vi "EFMC-7.vi"(0 "数组":u8[](array[numeric])) -> (1 "视速度增量":cluster{"X轴增量":i16, "Y轴增量":i16, "Z轴增量":i16}, 2 "姿态和速度增量有效性":T2, 3 "俯仰角速率":i16, 4 "滚转角速率":i16, 6 "角度增量":cluster{"X轴角增量":i16, "Y轴角增量":i16, "Z轴角增量":i16}, 8 "X轴过载":i16, 10 "偏航角速率":i16, 12 "Z轴过载":i16, 13 "角速率和过载有效性":T1, 14 "Y轴过载":i16)   [LabVIEW 2012]
uses:
  index-i16.vi
  XX-I16.vi
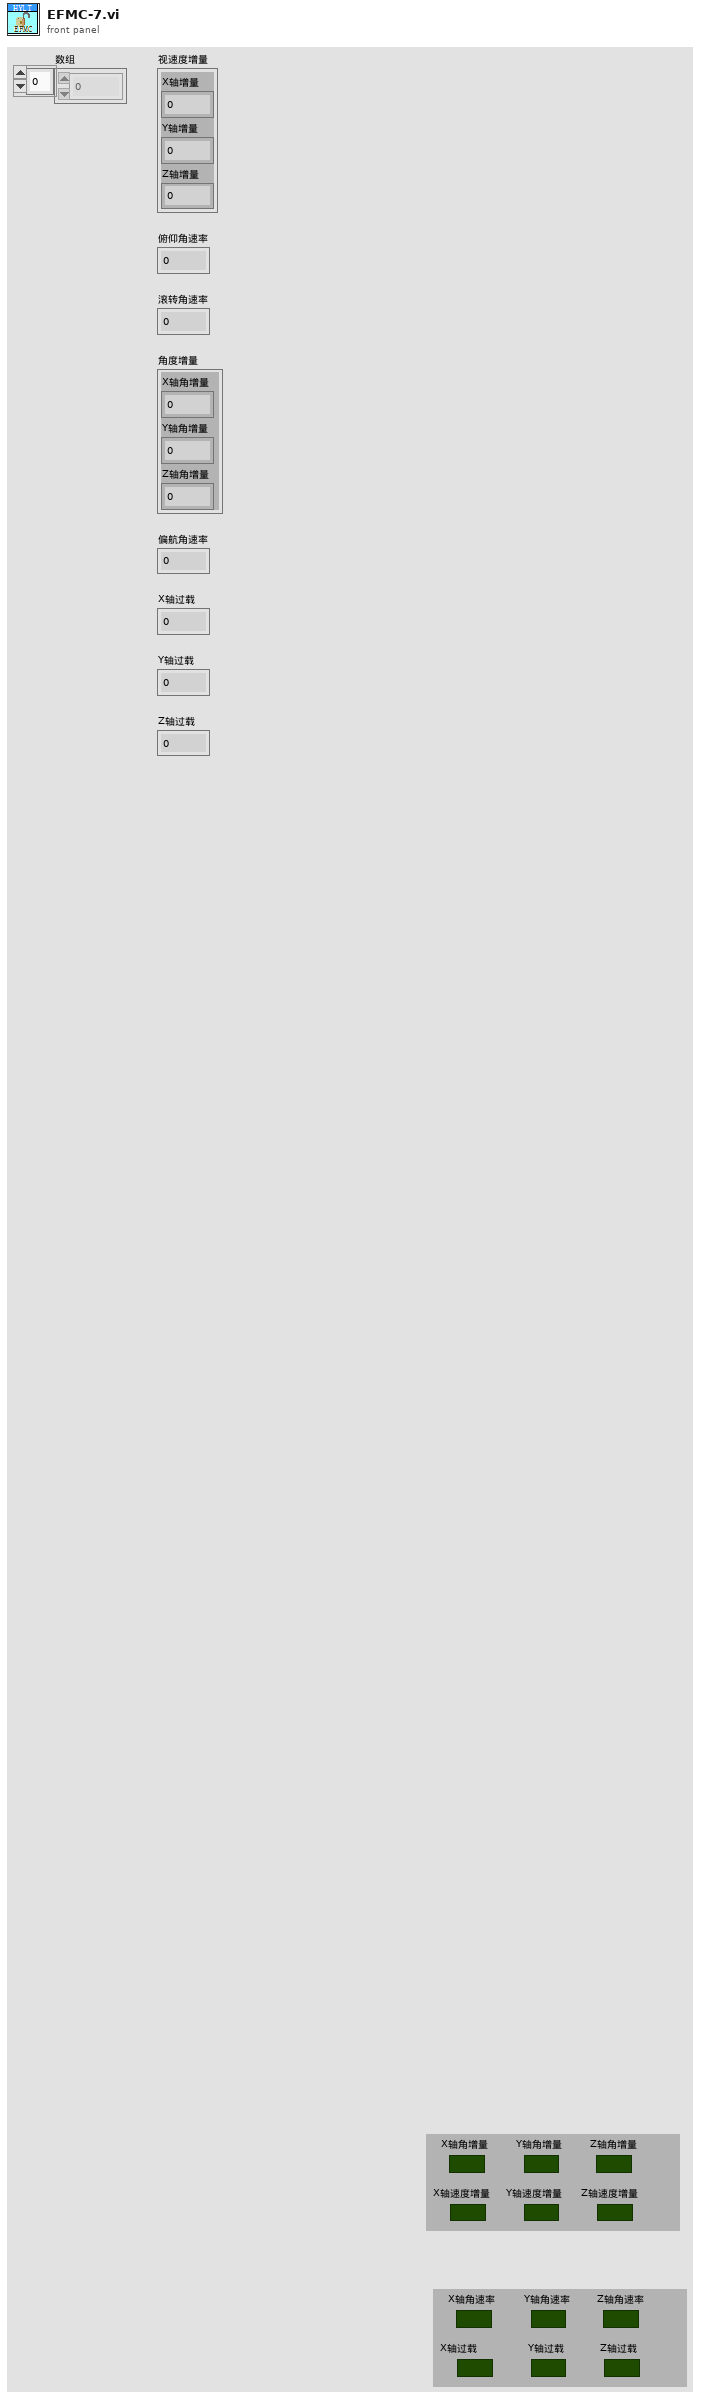
[diagram p1: front panel]
types:
  T1 = cluster{"X轴角速率":bool, "Y轴角速率":bool, "Z轴角速率":bool, "X轴过载":bool, "Y轴过载":bool, "Z轴过载":bool}
  T2 = cluster{"X轴角增量":bool, "Y轴角增量":bool, "Z轴角增量":bool, "X轴速度增量":bool, "Y轴速度增量":bool, "Z轴速度增量":bool}
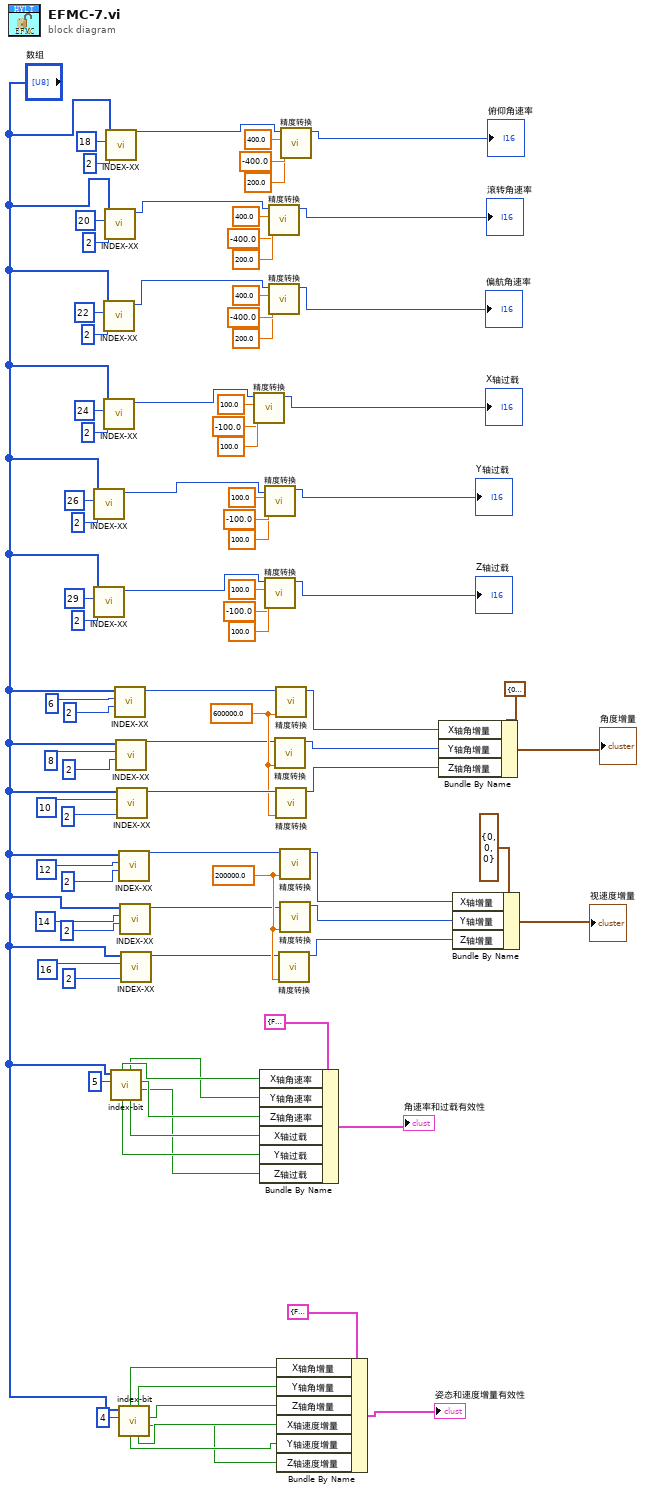
[diagram p0: block diagram]
diagram:
  w49 = 200000.0 ("单位")
  w40 = 600000.0 ("单位")
  n1 = call-poly "INDEX-XX.vi"("长度"=2, "索引"=26, "数组"="数组") -> ("数值输出"=w56:i16)  [unwired: 8 in]
  n2 = call-poly "INDEX-XX.vi"("长度"=2, "索引"=29, "数组"="数组") -> ("数值输出"=w51:i16)  [unwired: 8 in]
  n3 = call-poly "INDEX-XX.vi"("长度"=2, "索引"=22, "数组"="数组") -> ("数值输出"=w66:i16)  [unwired: 8 in]
  n4 = call-poly "INDEX-XX.vi"("长度"=2, "索引"=24, "数组"="数组") -> ("数值输出"=w61:i16)  [unwired: 8 in]
  n5 = call-poly "INDEX-XX.vi"("长度"=2, "索引"=20, "数组"="数组") -> ("数值输出"=w71:i16)  [unwired: 8 in]
  n6 = call-poly "INDEX-XX.vi"("长度"=2, "索引"=18, "数组"="数组") -> ("数值输出"=w76:i16)  [unwired: 8 in]
  n7 = call "index-bit.vi"("index"=5, "array"="数组") -> ("bit6"=w13:bool, "bit2"=w16:bool, "bit4"=w15:bool, "bit1"=w17:bool, "bit5"=w14:bool, "bit0"=w18:bool)  [unwired: 2 in, 2 out]
  n8 = call-poly "INDEX-XX.vi"("长度"=2, "索引"=6, "数组"="数组") -> ("数值输出"=w36:i16)  [unwired: 8 in]
  n9 = call-poly "INDEX-XX.vi"("长度"=2, "索引"=8, "数组"="数组") -> ("数值输出"=w38:i16)  [unwired: 8 in]
  n10 = call-poly "INDEX-XX.vi"("长度"=2, "索引"=10, "数组"="数组") -> ("数值输出"=w41:i16)  [unwired: 8 in]
  n11 = call-poly "INDEX-XX.vi"("长度"=2, "索引"=12, "数组"="数组") -> ("数值输出"=w43:i16)  [unwired: 8 in]
  n12 = call "index-bit.vi"("index"=4, "array"="数组") -> ("bit6"=w5:bool, "bit2"=w8:bool, "bit4"=w7:bool, "bit1"=w9:bool, "bit5"=w6:bool, "bit0"=w10:bool)  [unwired: 2 in, 2 out]
  n13 = call-poly "INDEX-XX.vi"("长度"=2, "索引"=14, "数组"="数组") -> ("数值输出"=w45:i16)  [unwired: 8 in]
  n14 = call-poly "INDEX-XX.vi"("长度"=2, "索引"=16, "数组"="数组") -> ("数值输出"=w47:i16)  [unwired: 8 in]
  n15 = call-poly "精度转换.vi"("单位"=100.0, "下限"=-100.0, "上限"=100.0, "数值输入"=w61) -> ("输出"=→"X轴过载":i16)  [unwired: 7 in]
  n16 = Bundle By Name(cluster=T1 {"X轴角速率"=FALSE, "Y轴角速率"=FALSE, "Z轴角速率"=FALSE, "X轴过载"=FALSE, "Y轴过载"=FALSE, "Z轴过载"=FALSE} ("姿态和速度增量有效性"), "X轴角速率"=w18, "Y轴角速率"=w17, "Z轴角速率"=w16, "X轴过载"=w15, "Y轴过载"=w14, "Z轴过载"=w13) -> (→"角速率和过载有效性":T1)
  n17 = call-poly "精度转换.vi"("单位"=100.0, "下限"=-100.0, "上限"=100.0, "数值输入"=w56) -> ("输出"=→"Y轴过载":i16)  [unwired: 7 in]
  n18 = call-poly "精度转换.vi"("单位"=100.0, "下限"=-100.0, "上限"=100.0, "数值输入"=w51) -> ("输出"=→"Z轴过载":i16)  [unwired: 7 in]
  n19 = call-poly "精度转换.vi"("单位"=200.0, "下限"=-400.0, "上限"=400.0, "数值输入"=w71) -> ("输出"=→"滚转角速率":i16)  [unwired: 7 in]
  n20 = call-poly "精度转换.vi"("单位"=200.0, "下限"=-400.0, "上限"=400.0, "数值输入"=w66) -> ("输出"=→"偏航角速率":i16)  [unwired: 7 in]
  n21 = call-poly "精度转换.vi"("单位"=w40, "数值输入"=w38) -> ("输出"=w39:i16)  [unwired: 9 in]
  n22 = call-poly "精度转换.vi"("单位"=w40, "数值输入"=w36) -> ("输出"=w37:i16)  [unwired: 9 in]
  n23 = call-poly "精度转换.vi"("单位"=w40, "数值输入"=w41) -> ("输出"=w42:i16)  [unwired: 9 in]
  n24 = Bundle By Name(cluster=T2 {"X轴角增量"=FALSE, "Y轴角增量"=FALSE, "Z轴角增量"=FALSE, "X轴速度增量"=FALSE, "Y轴速度增量"=FALSE, "Z轴速度增量"=FALSE} ("角速度和过载有效性"), "X轴角增量"=w10, "Y轴角增量"=w9, "Z轴角增量"=w8, "X轴速度增量"=w7, "Y轴速度增量"=w6, "Z轴速度增量"=w5) -> (→"姿态和速度增量有效性":T2)
  n25 = call-poly "精度转换.vi"("单位"=w49, "数值输入"=w47) -> ("输出"=w48:i16)  [unwired: 9 in]
  n26 = call-poly "精度转换.vi"("单位"=w49, "数值输入"=w43) -> ("输出"=w44:i16)  [unwired: 9 in]
  n27 = call-poly "精度转换.vi"("单位"=w49, "数值输入"=w45) -> ("输出"=w46:i16)  [unwired: 9 in]
  n28 = call-poly "精度转换.vi"("单位"=200.0, "下限"=-400.0, "上限"=400.0, "数值输入"=w76) -> ("输出"=→"俯仰角速率":i16)  [unwired: 7 in]
  n29 = Bundle By Name(cluster=cluster{"X轴角增量":i16, "Y轴角增量":i16, "Z轴角增量":i16} {"X轴角增量"=0, "Y轴角增量"=0, "Z轴角增量"=0} ("角度增量"), "X轴角增量"=w37, "Y轴角增量"=w39, "Z轴角增量"=w42) -> (→"角度增量":cluster{"X轴角增量":i16, "Y轴角增量":i16, "Z轴角增量":i16})
  n30 = Bundle By Name(cluster=cluster{"X轴增量":i16, "Y轴增量":i16, "Z轴增量":i16} {"X轴增量"=0, "Y轴增量"=0, "Z轴增量"=0} ("视速度增量"), "X轴增量"=w44, "Y轴增量"=w46, "Z轴增量"=w48) -> (→"视速度增量":cluster{"X轴增量":i16, "Y轴增量":i16, "Z轴增量":i16})
